vi "Target_gradient_calculation.vi"(0 "MD420.lvclass":refnum<class "MD420.lvclass">, 1 "PUMA 1/4":bool, 2 "Load change":bool, 3 "PG target Setpoint":dbl, 4 "ACT target value":dbl, 5 "SUM Ps":dbl, 6 "Ps Grad":dbl, 7 "error in":errorcluster, 9 "ACT Eff SP (k-1)":dbl) -> (20 "MD420.lvclass out":refnum<class "MD420.lvclass">, 23 "PG1":dbl, 24 "Target Grad":dbl, 27 "error out":errorcluster)   [LabVIEW 2022 SP3, in "MD420.lvclass"]
uses:
  MD420.lvclass
  MD420.lvclass/MD420.ctl
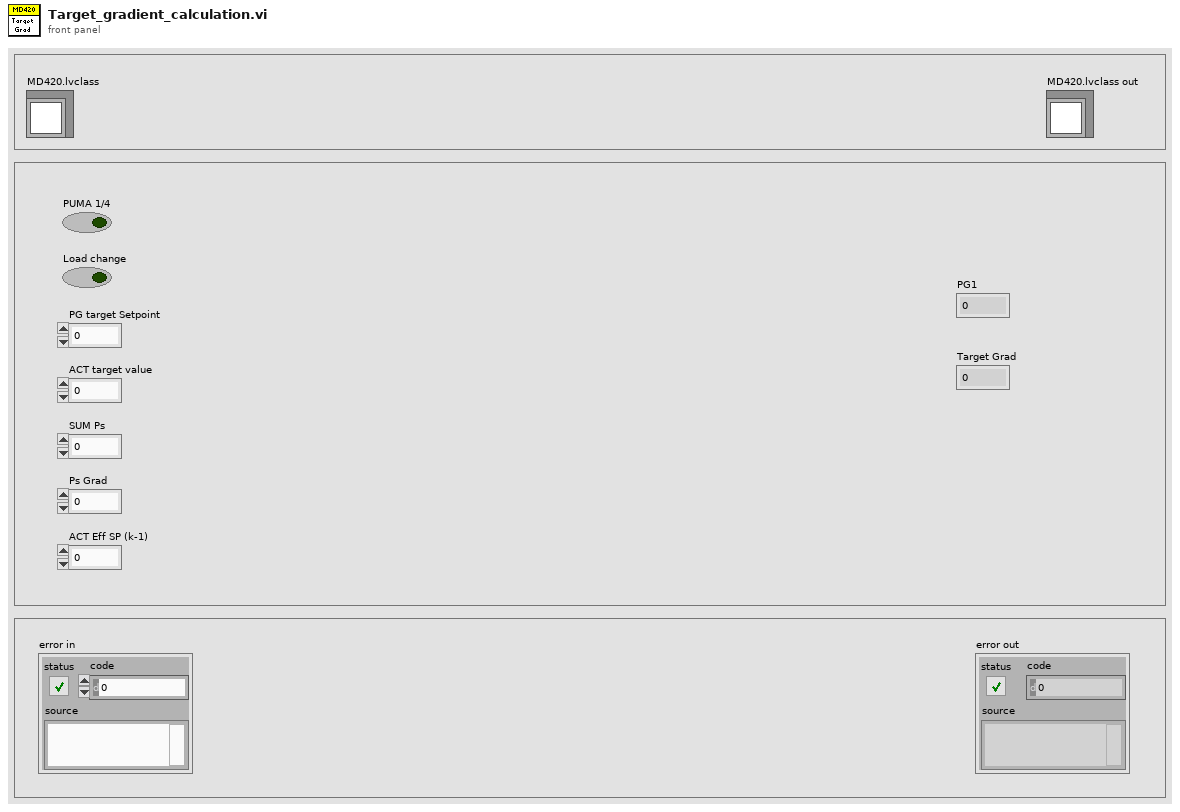
[diagram p1: front panel]
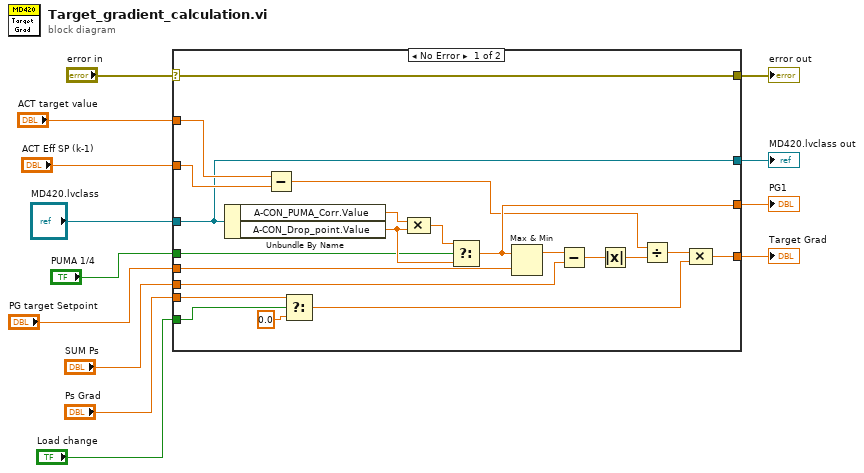
[diagram p0: block diagram]
diagram:
  n1 = case shown="No Error" "error in" {
    selector: "error in" -> [w15 w35]
    tunnel: "MD420.lvclass" -> [w14 _]
    tunnel: [w31 _] -> w11
    tunnel: "PUMA 1/4" -> [w28 _]
    tunnel: "PG target Setpoint" -> [w27 _]
    tunnel: "SUM Ps" -> [w26 _]
    tunnel: "ACT target value" -> [w24 _]
    tunnel: "ACT Eff SP (k-1)" -> [w23 _]
    tunnel: "Load change" -> [w21 _]
    tunnel: "Ps Grad" -> [w19 _]
    tunnel: [w16 _] -> w3
    tunnel: [w15 w35] -> w2
    tunnel: [w14 _] -> w1
    frame No Error {
      n2 = Unbundle By Name(w14) -> ("A-CON_PUMA_Corr.Value"=w34:dbl, "A-CON_Drop_point.Value"=w32:dbl)
      n3 = Subtract(x=w24, y=w23) -> (x-y=w22:dbl)
      n4 = Select(t=w19, s=w21, f=0.0) -> (s? t:f=w17:dbl)
      n5 = Compound Arithmetic op=MULTIPLY(w34, w32) -> (w33:dbl)
      n6 = Select(t=w33, s=w28, f=w32) -> (s? t:f=w31:dbl)
      n7 = Max & Min(x=w31, y=w27) -> (max(x,y)=w30:dbl)  [unwired: 1 out]
      n8 = Subtract(x=w30, y=w26) -> (x-y=w29:dbl)
      n9 = Absolute Value(x=w29) -> (abs(x)=w25:dbl)
      n10 = Divide(x=w22, y=w25) -> (x/y=w18:dbl)
      n11 = Compound Arithmetic op=MULTIPLY(w18, w17) -> (w16:dbl)
    }
    frame Error {
    }
  }
  "PG1" <- w11
  "Target Grad" <- w3
  "error out" <- w2
  "MD420.lvclass out" <- w1
